vi "Parsing Data.vi"(11 "String":string) -> (3 "Array":u8[][](array[numeric]))   [LabVIEW 2019, in "Day 15.lvlib"]
uses:
  Day 15.lvlib
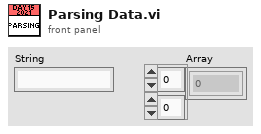
[diagram p1: front panel]
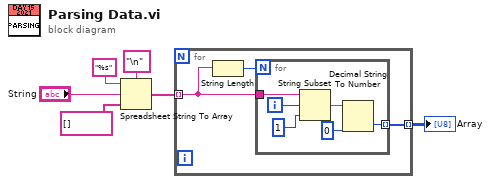
[diagram p0: block diagram]
diagram:
  n1 = Spreadsheet String To Array(delimiter (Tab)="\n", format string="%s", spreadsheet string="String", array type (2D Dbl)=string[] []) -> (array=w5:string[])
  n2 = for {
    tunnel: w5 -> [w9] mode=indexing
    tunnel: [w7] -> w6 mode=indexing
    n3 = String Length(string=w9) -> (length=w8:i32)
    n4 = for {
      N: w8 -> [_]
      tunnel: w9 -> [w15]
      tunnel: [w11] -> w7 mode=indexing
      i -> [w14]
      n5 = String Subset(string=w15, offset (0)=w14, length (rest)=1 ("length (rest)")) -> (substring=w12:string)
      n6 = Decimal String To Number(string=w12, default (0L)=u8 0 ("default (0 I32)")) -> (number=w11:u8)  [unwired: 1 in, 1 out]
    }
  }
  "Array" <- w6
